vi "Find Direction From Lidar.vi"(8 "error in (no error)":errorcluster, 11 "VISA resource name":refnum<visa-resource-name>) -> (0 "Go Straight":bool, 1 "Turn Left":bool, 2 "Turn Right":bool, 3 "VISA resource name out":refnum<visa-resource-name>, 4 "error out":errorcluster, 5 "Stop Robot":bool, 6 "Direction":dbl[](array[numeric]), 7 "Magnitude":dbl[](array[numeric]))   [LabVIEW 2011]
uses:
  <vilib>/robotics/Obstacle Avoidance/Simple Vector Field Histogram/Panic Range.ctl
  <vilib>/robotics/Obstacle Avoidance/Simple Vector Field Histogram/NI_Robotics_Simple Vector Field Histogram.lvlib
  <instrlib>/Hokuyo URG Series/Hokuyo URG Series.lvlib
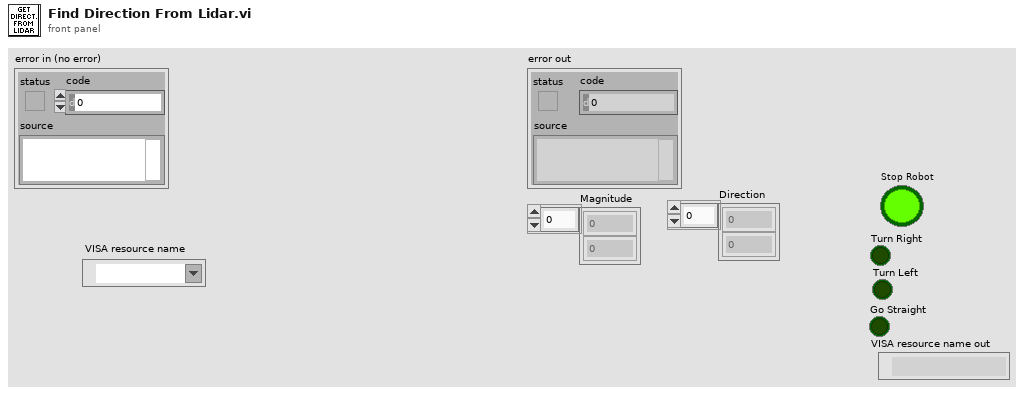
[diagram p1: front panel]
types:
  T1 = typedef "NI_Robotics_Simple Vector Field Histogram.lvlib/Panic Range.ctl" = cluster{"panic threshold distance (0)":dbl, "panic threshold angle (0)":dbl}
  T2 = typedef "NI_Robotics_Simple Vector Field Histogram.lvlib/Gap Description.ctl" = cluster{"angle to gap":dbl, "size of gap":dbl}
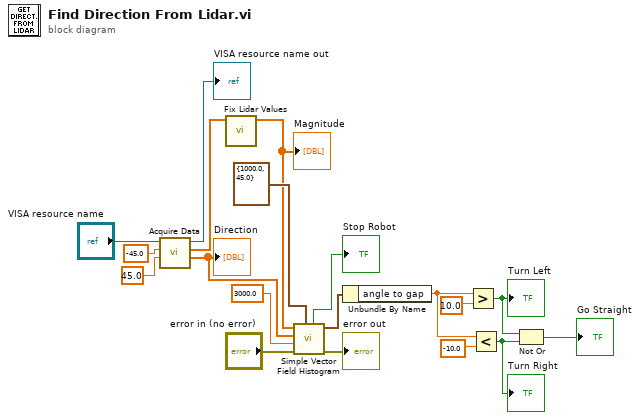
[diagram p0: block diagram]
diagram:
  n1 = call <instrlib>:"Acquire Data.vi"("End Point (120°)"=45.0, "Start Point (-120°)"=-45.0, "VISA resource name"="VISA resource name") -> ("Direction"=w3:dbl[], "Magnitude"=w1:dbl[], "VISA resource name out"=→"VISA resource name out":refnum<visa-resource-name>)  [unwired: 5 in, 1 out]
  "Direction" <- w3
  n2 = call "Fix Lidar Values.vi"("Distances In"=w1) -> ("Distances Out"=w2:dbl[])  [unwired: 10 in]
  "Magnitude" <- w2
  n3 = call <vilib>:"Simple Vector Field Histogram.vi"("panic range"=T1 {"panic threshold distance (0)"=1000.0, "panic threshold angle (0)"=45.0}, "error in (no error)"="error in (no error)", "distance threshold"=3000.0, "direction angles"=w3, "distances"=w2) -> ("error out"=→"error out":errorcluster, "largest gap"=w17:T2, "obstacle within panic range"=→"Stop Robot":bool)  [unwired: 2 in, 2 out]
  n4 = Unbundle By Name(w17) -> ("angle to gap"=w10:dbl)
  n5 = Greater?(x=w10, y=10.0) -> (0:w12:bool)
  "Turn Left" <- w12
  n6 = Less?(x=w10, y=-10.0) -> (x < y?=w11:bool)
  "Turn Right" <- w11
  n7 = Not Or(1:w11, 2:w12) -> (0:→"Go Straight":bool)
